vi "ConfigureHWSynced.vi"(0 "object in":refnum<class "Hamamatsu.lvclass">, 2 "FramesPerAquisionCycle":i32, 3 "CameraBufferSize":i32, 5 "error in (no error)":errorcluster) -> (14 "object out":refnum<class "Hamamatsu.lvclass">, 19 "error out":errorcluster)   [LabVIEW 2021, in "Hamamatsu.lvclass"]
uses:
  Hamamatsu.lvclass
  Hamamatsu.lvclass/Hamamatsu.ctl
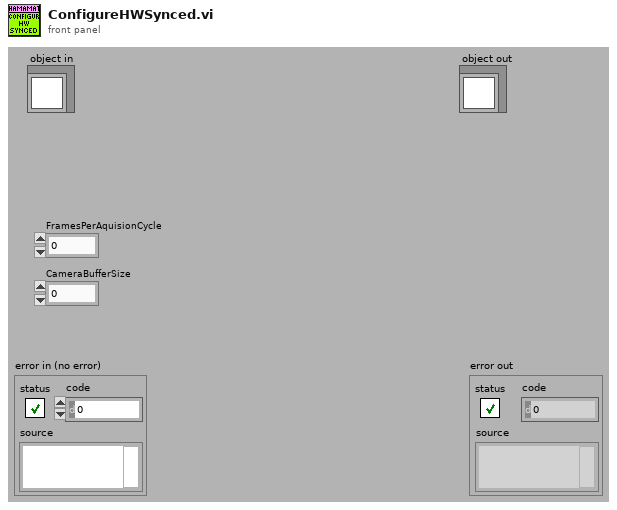
[diagram p1: front panel]
types:
  T1 = typedef "IMAQ Image.ctl" = refnum<image>
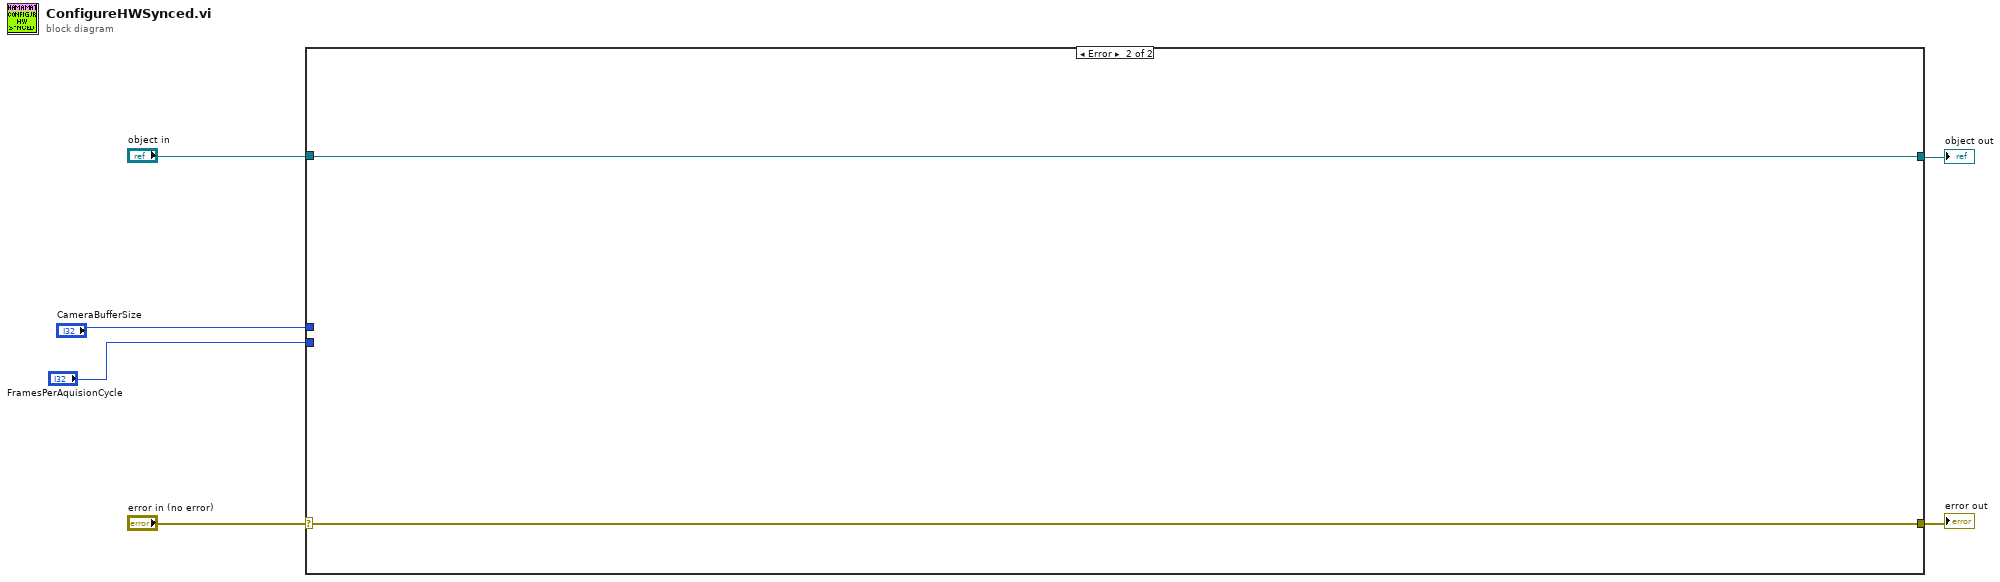
[diagram p0: block diagram]
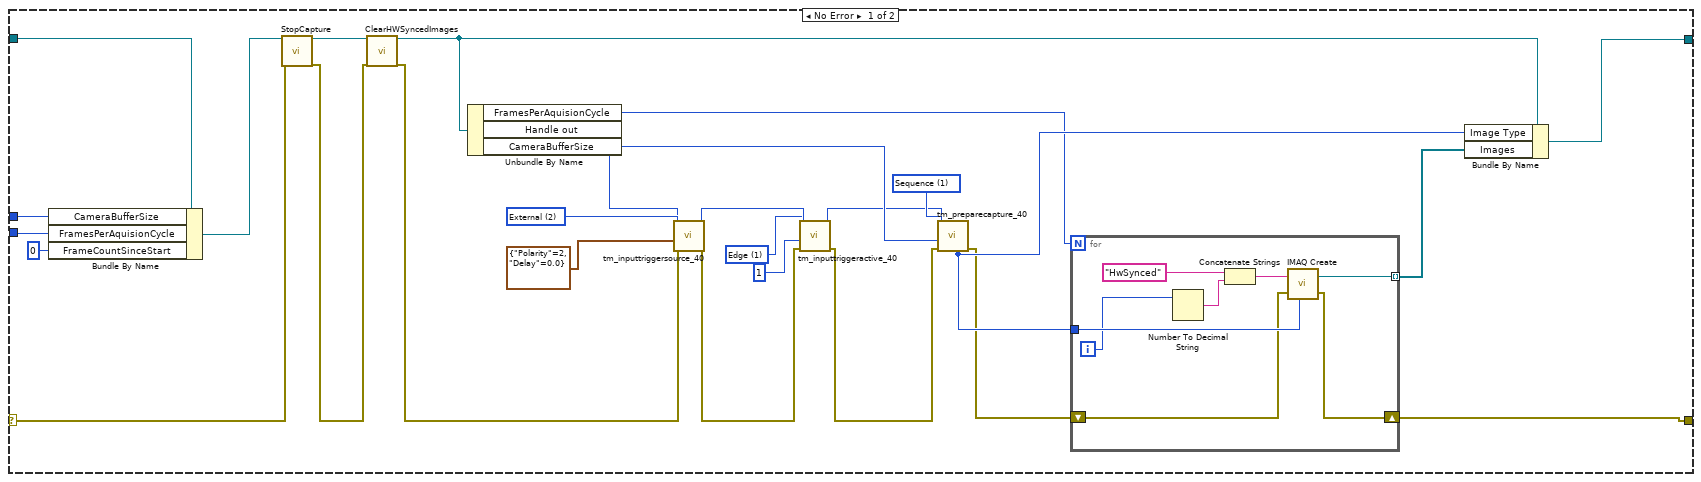
[diagram p2: hidden frame]
diagram:
  n1 = case shown="Error" "error in (no error)" {
    selector: "error in (no error)" -> [w8 w43]
    tunnel: [w28 w43] -> w5
    tunnel: [w29 w42] -> w3
    tunnel: "object in" -> [w13 w42]
    tunnel: "CameraBufferSize" -> [w12 _]
    tunnel: "FramesPerAquisionCycle" -> [w14 _]
    frame No Error {
      w22 = 1 items=["Edge"=1, "Level"=2, "Sync Readout"=3, "Point"=4] ("Active")
      w27 = 2 items=["Internal"=1, "External"=2, "Software"=3, "Master Pulse"=4] ("Source")
      w33 = 1 items=["Snap", "Sequence"] ("Capture mode")
      n2 = Bundle By Name(cluster=w13, "CameraBufferSize"=w12, "FramesPerAquisionCycle"=w14, "FrameCountSinceStart"=0) -> (w10:refnum<class "Hamamatsu.lvclass">)
      n3 = call-dynamic "StopCapture.vi"("object in"=w10, "error in (no error)"=w8) -> ("object out"=w9:refnum<class "Hamamatsu.lvclass">, "error out"=w7:errorcluster)  [unwired: 16 in]
      n4 = call-dynamic "ClearHWSyncedImages.vi"("object in"=w9, "error in (no error)"=w7) -> ("object out"=w17:refnum<class "Hamamatsu.lvclass">, "error out"=w16:errorcluster)  [unwired: 16 in]
      n5 = Unbundle By Name(w17) -> ("FramesPerAquisionCycle"=w15:i32, "Handle out"=w26:u32, "CameraBufferSize"=w30:i32)
      n6 = call <userlib>:"tm_inputtriggersource_40.vi"("error in (no error)"=w16, "External Options"=cluster{"Polarity":i32, "Delay":dbl} {"Polarity"=2, "Delay"=0.0}, "Source"=w27, "Handle in"=w26) -> ("error out"=w20:errorcluster, "Handle out"=w24:u32)  [unwired: 6 in]
      n7 = call <userlib>:"tm_inputtriggeractive_40.vi"("error in (no error)"=w20, "Times"=1, "Active"=w22, "Handle in"=w24) -> ("error out"=w19:errorcluster, "Handle out"=w23:u32)  [unwired: 6 in]
      n8 = call <userlib>:"tm_preparecapture_40.vi"("error in (no error)"=w19, "Frames"=w30, "Capture mode"=w33, "Handle in"=w23) -> ("error out"=w31:errorcluster, "Image type"=w32:u32)  [unwired: 4 in, 2 out]
      n9 = for {
        N: w15 -> [_]
        tunnel: w32 -> [w40]
        shift-right: [w38] -> w28
        shift-left: w31 -> [w39]
        tunnel: [w37] -> w18 mode=indexing
        i -> [w36]
        n10 = Number To Decimal String(number=w36) -> (decimal integer string=w34:string)  [unwired: 1 in]
        n11 = Concatenate Strings("HwSynced" ("Image Name"), w34) -> (w35:string)
        n12 = call "IMAQ Create"("Image Name"=w35, "Image Type"=w40, "error in (no error)"=w39) -> ("New Image"=w37:T1, "error out"=w38:errorcluster)  [unwired: 2 in]
      }
      n13 = Bundle By Name(cluster=w17, "Image Type"=w32, "Images"=w18) -> (w29:refnum<class "Hamamatsu.lvclass">)
    }
    frame Error {
    }
  }
  "error out" <- w5
  "object out" <- w3
